vi "Get Current LV Bitness.vi"() -> (3 "bitness":string)   [LabVIEW 2020]
doc: "This VI returns a string \"32\" or \"64\" depending upon the bitness of the current LabVIEW environment."
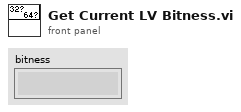
[diagram p1: front panel]
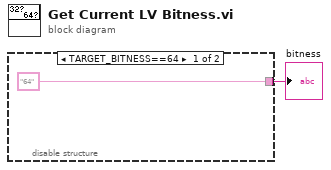
[diagram p0: block diagram]
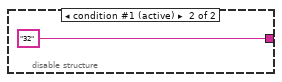
[diagram p2: hidden frame]
diagram:
  n1 = disable-structure shown="TARGET_BITNESS==64" {
    disable-tunnel: ["64" "32"] -> w1
    frame condition #0 {
    }
    frame condition #1 (active) {
    }
  }
  "bitness" <- w1
